vi "GetDataColumn.vi"(2 "TorqueUnit":string, 3 "Setting":T1={"TorqueSensor"={"Interface"="", "Read Unit"=enum."Kg.cm", "Encoder"=0, "Torque Filter"=0, "Max Torque"=2.0, "Max Power"=50.0, "Max Speed"=50.0, "Scale Factor CW"=2.0, "Scale Factor CCW"=2.0, "Scale Factor Zero"=2.0}, "TorqueSensorL"={"Interface"="", "Read Unit"=enum."Kg.cm", "Encoder"=0, "Torque Filter"=0, "Max Torque"=2.0, "Max Power"=50.0, "Max Speed"=50.0, "Scale Factor CW"=2.0, "Scale Factor CCW"=2.0, "Scale Factor Zero"=2.0}, "Power Meter"={"Wiring"=0, "Interface"="", "1P Mode"=1, "1P CurrentLimit"=0.0, "3P Mode"=1, "3P CurrentLimit"=0.0}, "Thermocouple"={"Interface"="", "value range"="T/C T type -100 ~ 400 degree C", "Channel Count"=8, "Limit 0"=0.0, "Limit 1"=0.0, "Limit 2"=0.0, "Limit 3"=0.0, "Limit 4"=0.0, "Limit 5"=0.0, "Limit 6"=0.0, "Limit 7"=0.0}, "DC-1000"={"Interface"=enum."AD-1"}, "ServoMotor"={"Interface"=enum."AD-1"}, "MotorDriver"={"D_Interface"="", "L_Interface"=""}, "TestMode"=enum."電子中軸測試", "PowerSupply"={"Interface"="", "Current"=50.0, "Voltage"=50.0}} {"Thermocouple"."Limit 7" format="%.1f"; "Thermocouple"."Limit 6" format="%.1f"; "Thermocouple"."Limit 5" format="%.1f"; "Thermocouple"."Limit 4" format="%.1f"; "Thermocouple"."Limit 3" format="%.1f"; "Thermocouple"."Limit 2" format="%.1f"; "Thermocouple"."Limit 1" format="%.1f"; "Thermocouple"."Limit 0" format="%.1f"; "Thermocouple"."Channel Count" min=0 max=24; "Power Meter"."3P Mode" items=["RMS", "MEAN", "DC"]; "Power Meter"."1P Mode" items=["RMS", "MEAN", "DC"]; "Power Meter"."Wiring" items=["1P2W", "1P2W+3P3W3M"]; "TorqueSensorL"."Scale Factor Zero" format="%#.6f"; "TorqueSensorL"."Scale Factor CCW" format="%#.6f"; "TorqueSensorL"."Scale Factor CW" format="%#.6f"; "TorqueSensorL"."Torque Filter" items=["OFF", "10Hz", "25Hz", "50Hz", "3Hz", "2Hz", "1Hz"]; "TorqueSensorL"."Encoder" items=["60-ppr"=60, "600-ppr"=600, "6000-ppr"=6000, "8192-ppr"=8192, "20-ppr"=20, "30-ppr"=30, "1-ppr"=1, "2-ppr"=2, "6-ppr"=6]; "TorqueSensor"."Scale Factor Zero" format="%#.6f"; "TorqueSensor"."Scale Factor CCW" format="%#.6f"; "TorqueSensor"."Scale Factor CW" format="%#.6f"; "TorqueSensor"."Torque Filter" items=["OFF", "10Hz", "25Hz", "50Hz", "3Hz", "2Hz", "1Hz"]; "TorqueSensor"."Encoder" items=["60-ppr"=60, "600-ppr"=600, "6000-ppr"=6000, "8192-ppr"=8192, "20-ppr"=20, "30-ppr"=30, "1-ppr"=1, "2-ppr"=2, "6-ppr"=6]}) -> (0 "TorqueIdx":u16[](array[numeric]), 1 "DataColumn":string[](array[string]))   [LabVIEW 2024]
uses:
  MFActor/SystemSettings.ctl
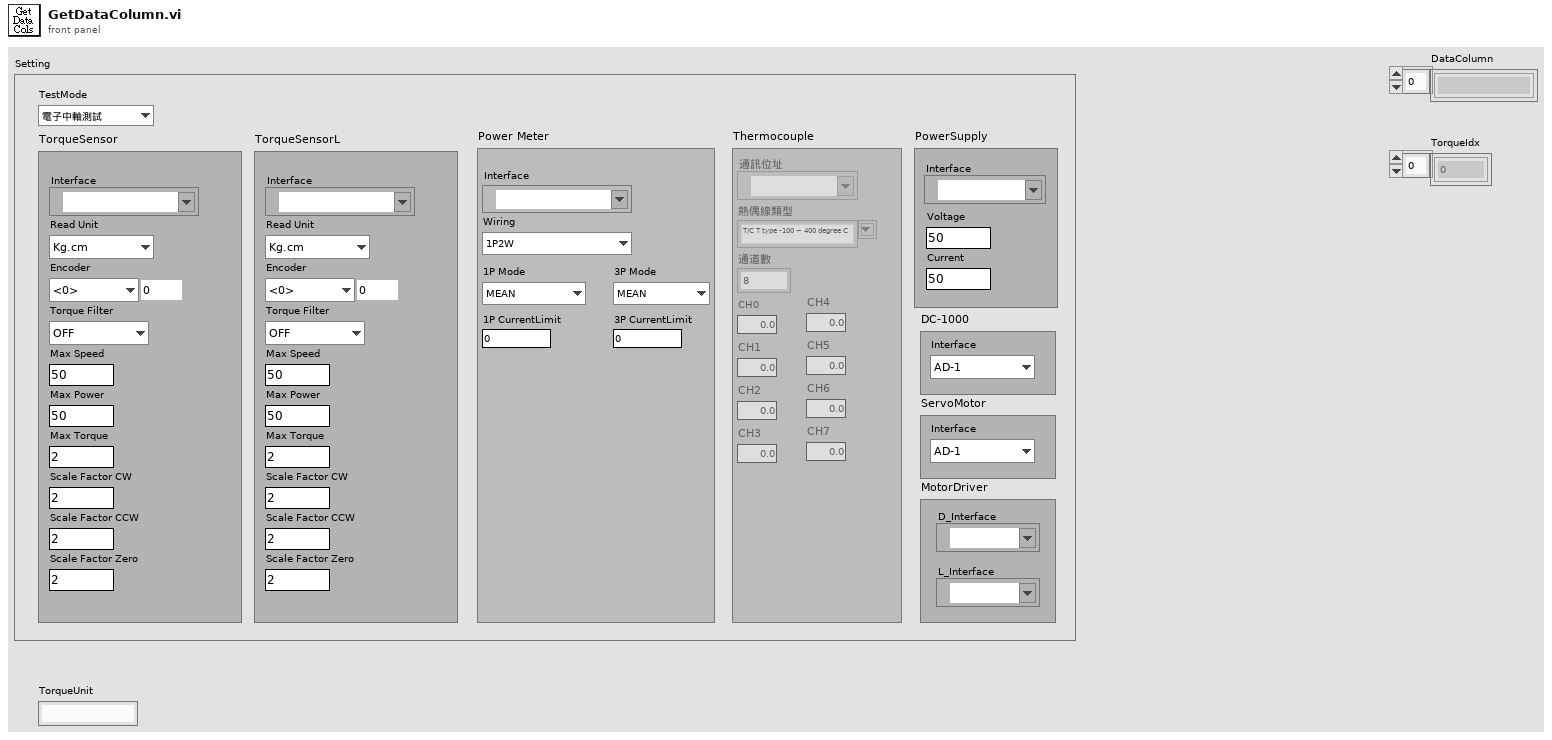
[diagram p1: front panel]
types:
  T1 = typedef "SystemSettings.ctl" = cluster{"TorqueSensor":cluster{"Interface":refnum<visa-resource-name>, "Read Unit":enum16{"oz.in", "oz.ft", "lb.in", "lb.ft", "g.cm", "Kg.cm", "mN.m", "cN.m", "N.m"}, "Encoder":u16, "Torque Filter":u16, "Max Torque":dbl, "Max Power":dbl, "Max Speed":dbl, "Scale Factor CW":dbl, "Scale Factor CCW":dbl, "Scale Factor Zero":dbl}, "TorqueSensorL":cluster{"Interface":refnum<visa-resource-name>, "Read Unit":enum16{"oz.in", "oz.ft", "lb.in", "lb.ft", "g.cm", "Kg.cm", "mN.m", "cN.m", "N.m"}, "Encoder":u16, "Torque Filter":u16, "Max Torque":dbl, "Max Power":dbl, "Max Speed":dbl, "Scale Factor CW":dbl, "Scale Factor CCW":dbl, "Scale Factor Zero":dbl}, "Power Meter":cluster{"Wiring":u16, "Interface":refnum<visa-resource-name>, "1P Mode":u16, "1P CurrentLimit":dbl, "3P Mode":u16, "3P CurrentLimit":dbl}, "Thermocouple":cluster{"Interface":refnum<visa-resource-name>, "value range":string, "Channel Count":i32, "Limit 0":dbl, "Limit 1":dbl, "Limit 2":dbl, "Limit 3":dbl, "Limit 4":dbl, "Limit 5":dbl, "Limit 6":dbl, "Limit 7":dbl}, "DC-1000":cluster{"Interface":enum16{"AD-0", "AD-1"}}, "ServoMotor":cluster{"Interface":enum16{"AD-0", "AD-1"}}, "MotorDriver":cluster{"D_Interface":refnum<visa-resource-name>, "L_Interface":refnum<visa-resource-name>}, "TestMode":enum16{"電子中軸測試", "中置電機測試"}, "PowerSupply":cluster{"Interface":refnum<visa-resource-name>, "Current":dbl, "Voltage":dbl}}
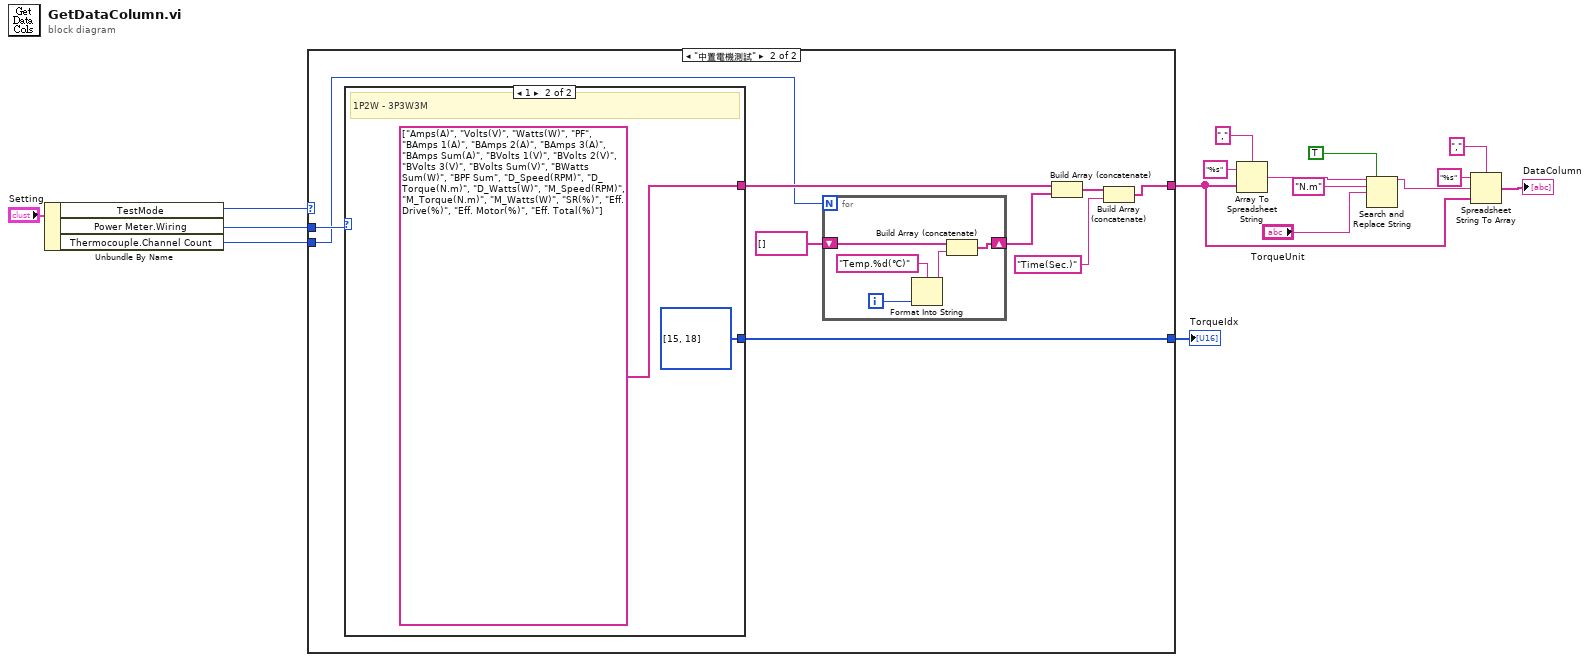
[diagram p0: block diagram]
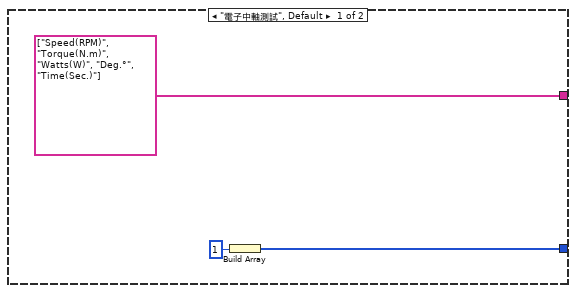
[diagram p2: hidden frame]
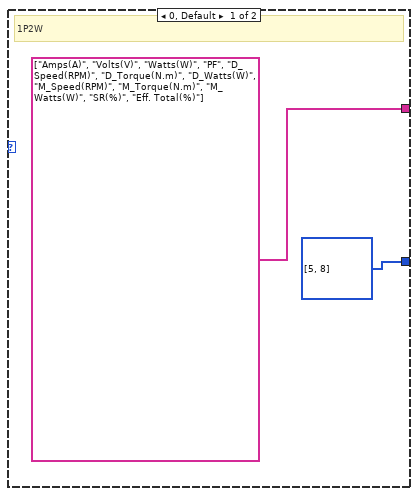
[diagram p3: hidden frame]
diagram:
  n1 = Unbundle By Name("Setting") -> ("TestMode"=w15:enum16{"電子中軸測試", "中置電機測試"}, "Power Meter.Wiring"=w13:u16, "Thermocouple.Channel Count"=w1:i32)
  n2 = case shown="\"中置電機測試\"" w15 {
    tunnel: [string[] ["Speed(RPM)", "Torque(N.m)", "Watts(W)", "Deg.°", "Time(Sec.)"] ("Strings []") w20] -> w3
    tunnel: [w17 w27] -> w14
    tunnel: w13 -> [_ w28]
    tunnel: w1 -> [_ w23]
    frame "電子中軸測試", Default {
      n3 = Build Array(u16 1) -> (w17:u16[])
    }
    frame "中置電機測試" {
      n4 = case shown="1" w28 {
        tunnel: [string[] ["Amps(A)", "Volts(V)", "Watts(W)", "PF", "D_Speed(RPM)", "D_Torque(N.m)", "D_Watts(W)", "M_Speed(RPM)", "M_Torque(N.m)", "M_Watts(W)", "SR(%)", "Eff. Total(%)"] string[] ["Amps(A)", "Volts(V)", "Watts(W)", "PF", "BAmps 1(A)", "BAmps 2(A)", "BAmps 3(A)", "BAmps Sum(A)", "BVolts 1(V)", "BVolts 2(V)", "BVolts 3(V)", "BVolts Sum(V)", "BWatts Sum(W)", "BPF Sum", "D_Speed(RPM)", "D_Torque(N.m)", "D_Watts(W)", "M_Speed(RPM)", "M_Torque(N.m)", "M_Watts(W)", "SR(%)", "Eff. Drive(%)", "Eff. Motor(%)", "Eff. Total(%)"]] -> w26
        tunnel: [u16[] [5, 8] u16[] [15, 18]] -> w27
        frame 0, Default {
          # "1P2W"
        }
        frame 1 {
          # "1P2W - 3P3W3M"
        }
      }
      n5 = for {
        N: w23 -> [_]
        shift-right: [w29] -> w24
        shift-left: string[] [] -> [w31]
        i -> [w32]
        n6 = Format Into String(format string="Temp.%d(℃)", w32) -> (resulting string=w30:string)  [unwired: 2 in, 1 out]
        n7 = Build Array (concatenate)(w31, w30) -> (w29:string[])
      }
      n8 = Build Array (concatenate)(w26, w24) -> (w22:string[])
      n9 = Build Array (concatenate)(w22, "Time(Sec.)") -> (w20:string[])
    }
  }
  "TorqueIdx" <- w14
  n10 = Array To Spreadsheet String(delimiter (Tab)=",", array=w3, 3:"%s" ("format string")) -> (spreadsheet string=w6:string)
  n11 = Search and Replace String(replace all?=TRUE ("replace all? (F)"), input string=w6, search string="N.m", replace string="TorqueUnit") -> (result string=w4:string)  [unwired: 4 in, 3 out]
  n12 = Spreadsheet String To Array(delimiter (Tab)=",", format string="%s", spreadsheet string=w4, array type (2D Dbl)=w3) -> (array=→"DataColumn":string[])
